vi "Globalt0.vi"() -> ()   [LabVIEW 2018]
panel:
  in  "current time":timestamp
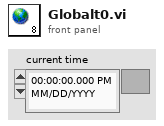
[diagram p1: front panel]
diagram:
